vi "ResetInit.vi"(8 "error in":errorcluster) -> (0 "error out":errorcluster)   [LabVIEW 2017]
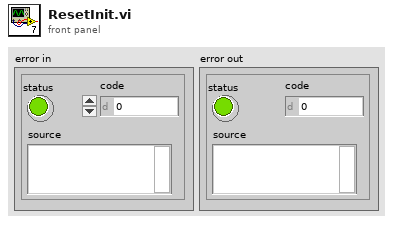
[diagram p1: front panel]
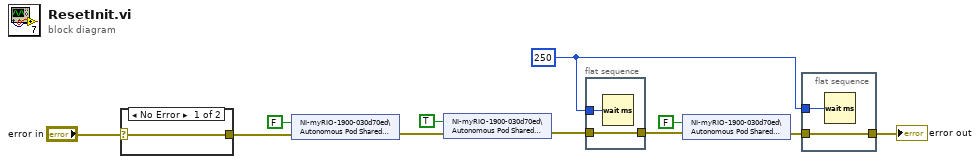
[diagram p0: block diagram]
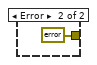
[diagram p2: hidden frame]
diagram:
  w7 = u32 250 ("milliseconds to wait")
  n1 = case shown="No Error" "error in" {
    selector: "error in" -> [w12 _]
    tunnel: [w12 errorcluster {"status"=FALSE, "code"=0, "source"=""} ("error in 2")] -> w2
    frame No Error {
    }
    frame Error {
    }
  }
  n2 = shared-variable "NI-myRIO-1900-030d70ed\\Autonomous Pod Shared Variables.lvlib\\ResetSensor"(FALSE ("ResetSensor"), error in=w2) -> (error out=w9:errorcluster)
  n3 = shared-variable "NI-myRIO-1900-030d70ed\\Autonomous Pod Shared Variables.lvlib\\SensePower"(TRUE ("SensePower"), error in=w9) -> (error out=w6:errorcluster)
  n4 = flat-sequence {
    tunnel: w7 -> [w15]
    tunnel: w6 -> [w14]
    tunnel: [w14] -> w5
    frame #0 {
      n5 = Wait (ms)(milliseconds to wait=w15) -> ()  [unwired: 1 out]
    }
  }
  n6 = shared-variable "NI-myRIO-1900-030d70ed\\Autonomous Pod Shared Variables.lvlib\\SensePower"(FALSE ("SensePower"), error in=w5) -> (error out=w3:errorcluster)
  n7 = flat-sequence {
    tunnel: w7 -> [w17]
    tunnel: [w16] -> w4
    tunnel: w3 -> [w16]
    frame #0 {
      n8 = Wait (ms)(milliseconds to wait=w17) -> ()  [unwired: 1 out]
    }
  }
  "error out" <- w4
